vi "Maximum Power.vi"(9 "Current (Amps) vs Voltage (Volts)":cluster{"voltage":dbl[], "current":dbl[]}(graph)) -> (2 "Maximum Power":dbl, 3 "Power (Watts) vs Voltage (Volts)":cluster{"voltage":dbl[], dbl[]}(graph), 4 "Current at Pmax":dbl, 6 "Voltage at Pmax":dbl)   [LabVIEW 2016]
panel:
  out "Current":dbl[](array[numeric])
  out "Voltage":dbl[](array[numeric])
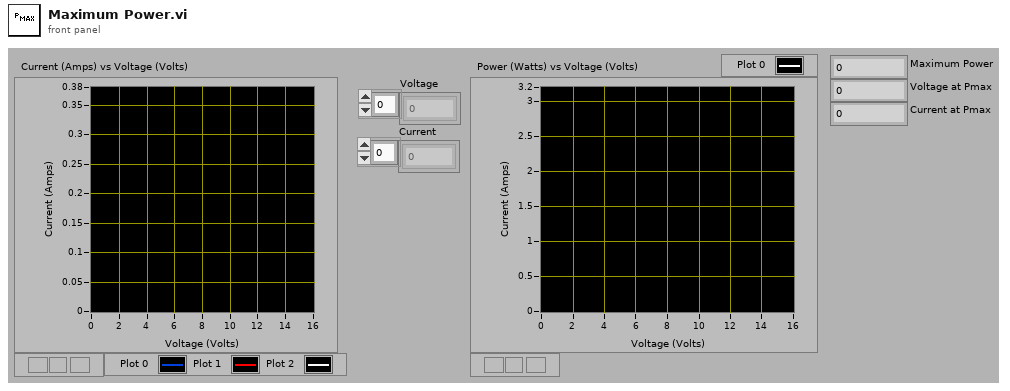
[diagram p1: front panel]
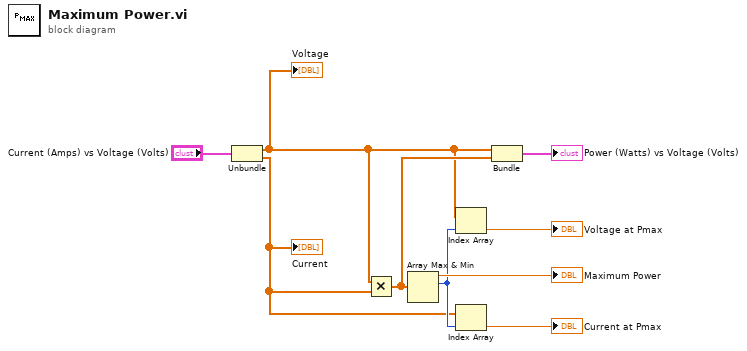
[diagram p0: block diagram]
diagram:
  n1 = Unbundle("Current (Amps) vs Voltage (Volts)") -> ("voltage"=w4:dbl[], "current"=w3:dbl[])
  "Voltage" <- w4
  "Current" <- w3
  n2 = Multiply(x=w4, y=w3) -> (x*y=w7:dbl[])
  n3 = Array Max & Min(array=w7) -> (max value=→"Maximum Power":dbl, max index (indices)=w8:i32)  [unwired: 2 out]
  n4 = Index Array(array=w4, index=w8) -> (element=→"Voltage at Pmax":dbl)
  n5 = Index Array(array=w3, index=w8) -> (element=→"Current at Pmax":dbl)
  n6 = Bundle("voltage"=w4, w7) -> (→"Power (Watts) vs Voltage (Volts)":cluster{"voltage":dbl[], dbl[]})  [unwired: 1 out]
